vi "Write Measurement Description Dictionary.vi"(8 "error in (no error)":errorcluster, 10 "NI Generic Parser.lvlib:Multi Step Database":refnum<class "Multi Step Database.lvclass">, 11 "NI Generic Parser in":refnum<class "NI Generic Parser.lvclass">) -> (0 "error out":errorcluster, 3 "NI Generic Parser out":refnum<class "NI Generic Parser.lvclass">)   [LabVIEW 2016, in "NI Generic Parser.lvlib" / "NI Generic Parser.lvclass"]
uses:
  NI Generic Parser.lvclass
  Support/Step Sequence Database/Multi Step Database.lvclass
  NI Generic Parser.lvclass/NI Generic Parser.ctl
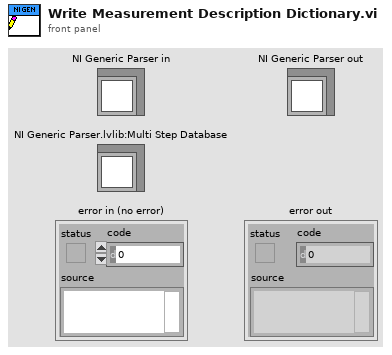
[diagram p1: front panel]
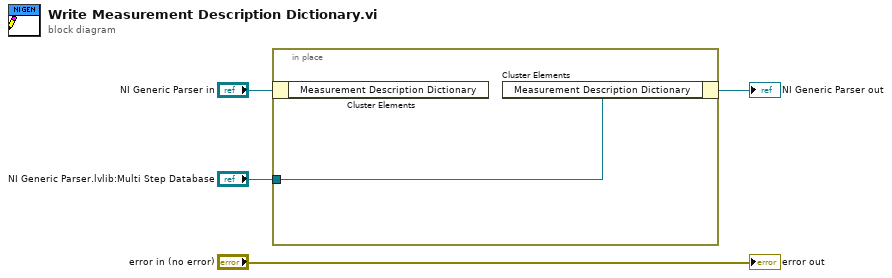
[diagram p0: block diagram]
diagram:
  n1 = in-place {
    in-place-border: "NI Generic Parser.lvlib:Multi Step Database" -> [w5]
    n2 = in-place-cluster #1("NI Generic Parser in") -> ()  [unwired: 1 out]
    n3 = in-place-cluster #1("Measurement Description Dictionary"=w5) -> (→"NI Generic Parser out":refnum<class "NI Generic Parser.lvclass">)
  }
  "error out" <- "error in (no error)"
